vi "Step.GetProperties.vi"(11 "String in":string) -> (1 "Warning":string, 2 "Parameters":dbl[](array[numeric]), 3 "Step":T1)   [LabVIEW 2013, in "Simple Sequence Tools - Shared.lvlib"]
uses:
  Simple Sequence Tools - Shared.lvlib
  Types/Step.Types.ctl
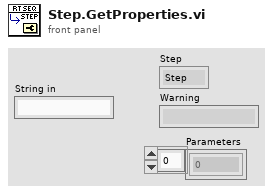
[diagram p1: front panel]
types:
  T1 = typedef "Simple Sequence Tools - Shared.lvlib/Step.Types.ctl" = enum8{"Step", "iStep", "Ramp", "Unchanged", "Unknown", "Sine", "LogSine", "LinearSine", "ForcedRamp", "SquareWave"}
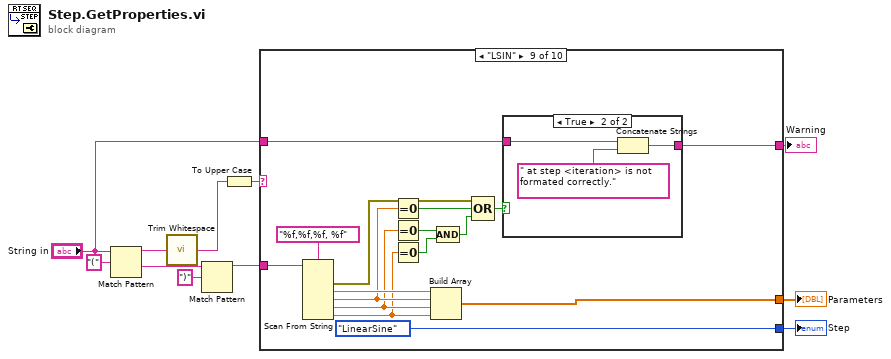
[diagram p0: block diagram]
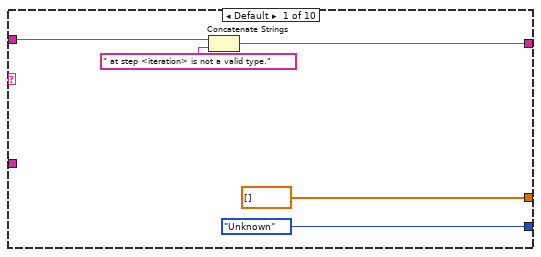
[diagram p2: hidden frame]
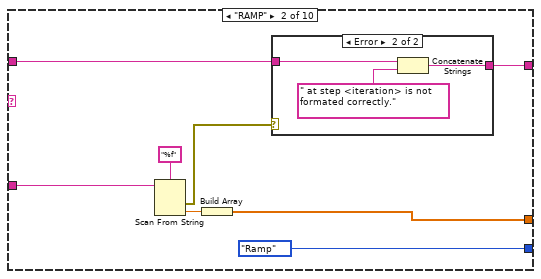
[diagram p3: hidden frame]
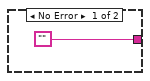
[diagram p4: hidden frame]
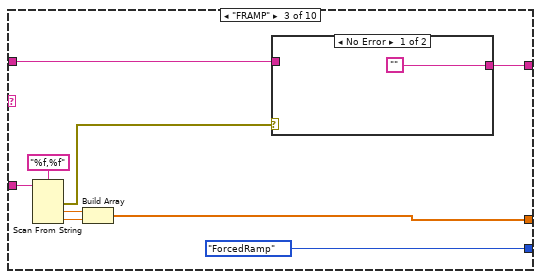
[diagram p5: hidden frame]
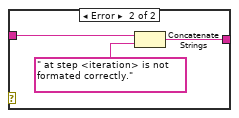
[diagram p6: hidden frame]
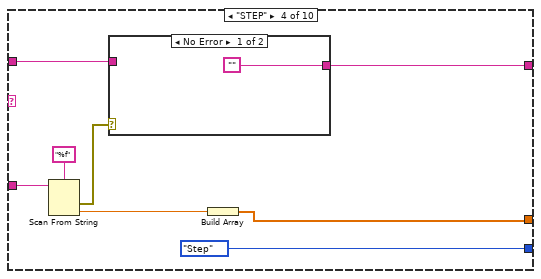
[diagram p7: hidden frame]
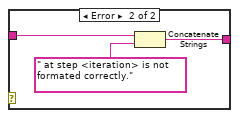
[diagram p8: hidden frame]
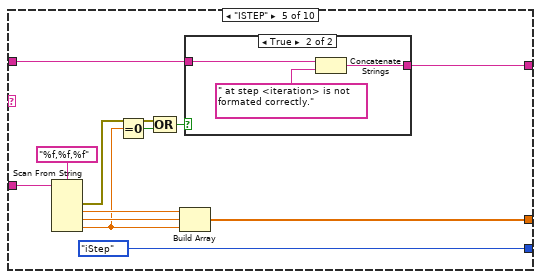
[diagram p9: hidden frame]
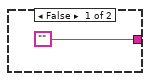
[diagram p10: hidden frame]
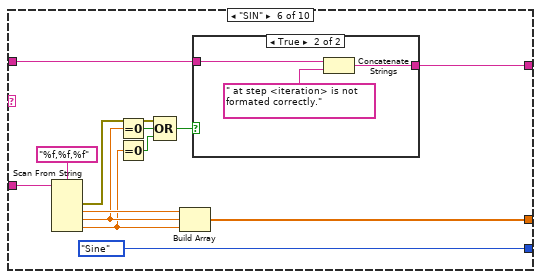
[diagram p11: hidden frame]
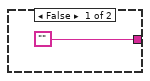
[diagram p12: hidden frame]
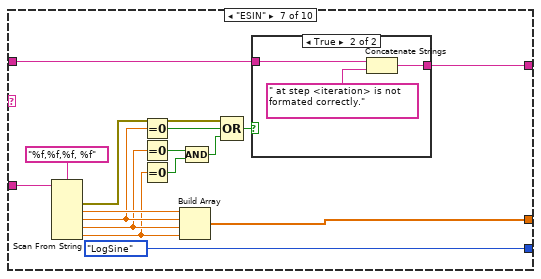
[diagram p13: hidden frame]
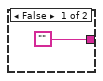
[diagram p14: hidden frame]
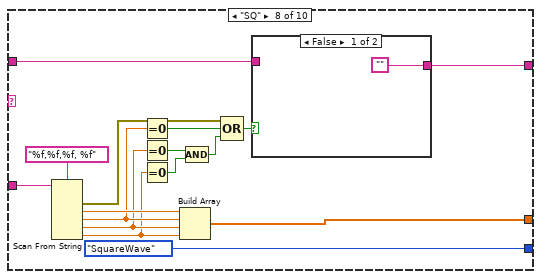
[diagram p15: hidden frame]
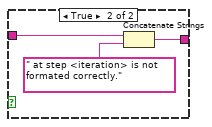
[diagram p16: hidden frame]
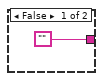
[diagram p17: hidden frame]
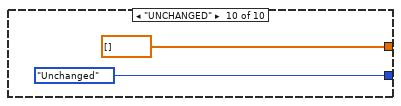
[diagram p18: hidden frame]
diagram:
  n1 = Match Pattern(string="String in", regular expression="(") -> (before substring=w8:string, after substring=w9:string)  [unwired: 1 in, 2 out]
  n2 = call <vilib>:"Trim Whitespace.vi"("string"=w8) -> ("trimmed string"=w11:string)  [unwired: 1 in]
  n3 = Match Pattern(string=w9, regular expression=")") -> (before substring=w4:string)  [unwired: 1 in, 3 out]
  n4 = To Upper Case(1:w11) -> (0:w6:string)
  n5 = case shown="\"LSIN\"" w6 {
    tunnel: [Step.Types."Unknown" Step.Types."Ramp" Step.Types."ForcedRamp" Step.Types."Step" Step.Types."iStep" Step.Types."Sine" Step.Types."LogSine" Step.Types."SquareWave" Step.Types."LinearSine" Step.Types."Unchanged"] -> w5
    tunnel: w4 -> [_ w19 w32 w48 w62 w79 w99 w119 w139 _]
    tunnel: [dbl[] [] w23 w29 w45 w60 w78 w98 w118 w138 dbl[] []] -> w3
    tunnel: "String in" -> [w14 w21 w35 w43 w58 w76 w96 w116 w136 _]
    tunnel: [w12 w20 w34 w42 w57 w75 w95 w115 w135 _] -> w1
    frame Default {
      n6 = Concatenate Strings(w14, " at step <iteration> is not a valid type.") -> (w12:string)
    }
    frame "RAMP" {
      n7 = Scan From String(format string="%f", input string=w19) -> (error out=w22:errorcluster, output 1=w17:dbl)  [unwired: 3 in, 2 out]
      n8 = Build Array(w17) -> (w23:dbl[])
      n9 = case shown="Error" w22 {
        tunnel: w21 -> [_ w27]
        tunnel: ["" w26] -> w20
        frame No Error {
        }
        frame Error {
          n10 = Concatenate Strings(w27, " at step <iteration> is not formated correctly.") -> (w26:string)
        }
      }
    }
    frame "FRAMP" {
      n11 = Scan From String(format string="%f,%f", input string=w32) -> (error out=w36:errorcluster, output 1=w30:dbl, output 2=w31:dbl)  [unwired: 4 in, 2 out]
      n12 = Build Array(w30, w31) -> (w29:dbl[])
      n13 = case shown="No Error" w36 {
        tunnel: w35 -> [_ w40]
        tunnel: ["" w39] -> w34
        frame No Error {
        }
        frame Error {
          n14 = Concatenate Strings(w40, " at step <iteration> is not formated correctly.") -> (w39:string)
        }
      }
    }
    frame "STEP" {
      n15 = Scan From String(format string="%f", input string=w48) -> (error out=w44:errorcluster, output 1=w46:dbl)  [unwired: 3 in, 2 out]
      n16 = case shown="No Error" w44 {
        tunnel: w43 -> [_ w52]
        tunnel: ["" w51] -> w42
        frame No Error {
        }
        frame Error {
          n17 = Concatenate Strings(w52, " at step <iteration> is not formated correctly.") -> (w51:string)
        }
      }
      n18 = Build Array(w46) -> (w45:dbl[])
    }
    frame "ISTEP" {
      n19 = Scan From String(format string="%f,%f,%f", input string=w62) -> (error out=w59:errorcluster, output 1=w63:dbl, output 2=w61:dbl, output 3=w55:dbl)  [unwired: 5 in, 2 out]
      n20 = Equal To 0?(x=w55) -> (x = 0?=w54:bool)
      n21 = Compound Arithmetic op=OR(w59, w54) -> (w56:bool)
      n22 = Build Array(w63, w61, w55) -> (w60:dbl[])
      n23 = case shown="True" w56 {
        tunnel: w58 -> [_ w68]
        tunnel: ["" w67] -> w57
        frame False {
        }
        frame True {
          n24 = Concatenate Strings(w68, " at step <iteration> is not formated correctly.") -> (w67:string)
        }
      }
    }
    frame "SIN" {
      n25 = Scan From String(format string="%f,%f,%f", input string=w79) -> (error out=w77:errorcluster, output 1=w80:dbl, output 2=w72:dbl, output 3=w71:dbl)  [unwired: 5 in, 2 out]
      n26 = Equal To 0?(x=w72) -> (x = 0?=w73:bool)
      n27 = Equal To 0?(x=w71) -> (x = 0?=w70:bool)
      n28 = Compound Arithmetic op=OR(w77, w73, w70) -> (w74:bool)
      n29 = Build Array(w80, w72, w71) -> (w78:dbl[])
      n30 = case shown="True" w74 {
        tunnel: w76 -> [_ w85]
        tunnel: ["" w84] -> w75
        frame False {
        }
        frame True {
          n31 = Concatenate Strings(w85, " at step <iteration> is not formated correctly.") -> (w84:string)
        }
      }
    }
    frame "ESIN" {
      n32 = Scan From String(format string="%f,%f,%f, %f", input string=w99) -> (error out=w97:errorcluster, output 1=w100:dbl, output 2=w92:dbl, output 3=w91:dbl, output 4=w90:dbl)  [unwired: 6 in, 2 out]
      n33 = Equal To 0?(x=w92) -> (x = 0?=w93:bool)
      n34 = Equal To 0?(x=w91) -> (x = 0?=w88:bool)
      n35 = Equal To 0?(x=w90) -> (x = 0?=w89:bool)
      n36 = Build Array(w100, w92, w91, w90) -> (w98:dbl[])
      n37 = Compound Arithmetic op=AND(w88, w89) -> (w87:bool)
      n38 = Compound Arithmetic op=OR(w97, w93, w87) -> (w94:bool)
      n39 = case shown="True" w94 {
        tunnel: w96 -> [_ w105]
        tunnel: ["" w104] -> w95
        frame False {
        }
        frame True {
          n40 = Concatenate Strings(w105, " at step <iteration> is not formated correctly.") -> (w104:string)
        }
      }
    }
    frame "SQ" {
      n41 = Scan From String(format string="%f,%f,%f, %f", input string=w119) -> (error out=w117:errorcluster, output 1=w120:dbl, output 2=w112:dbl, output 3=w111:dbl, output 4=w110:dbl)  [unwired: 6 in, 2 out]
      n42 = Equal To 0?(x=w112) -> (x = 0?=w113:bool)
      n43 = Equal To 0?(x=w111) -> (x = 0?=w108:bool)
      n44 = Equal To 0?(x=w110) -> (x = 0?=w109:bool)
      n45 = Build Array(w120, w112, w111, w110) -> (w118:dbl[])
      n46 = Compound Arithmetic op=AND(w108, w109) -> (w107:bool)
      n47 = Compound Arithmetic op=OR(w117, w113, w107) -> (w114:bool)
      n48 = case shown="False" w114 {
        tunnel: w116 -> [_ w125]
        tunnel: ["" w124] -> w115
        frame False {
        }
        frame True {
          n49 = Concatenate Strings(w125, " at step <iteration> is not formated correctly.") -> (w124:string)
        }
      }
    }
    frame "LSIN" {
      n50 = Scan From String(format string="%f,%f,%f, %f", input string=w139) -> (error out=w137:errorcluster, output 1=w140:dbl, output 2=w132:dbl, output 3=w131:dbl, output 4=w130:dbl)  [unwired: 6 in, 2 out]
      n51 = Equal To 0?(x=w132) -> (x = 0?=w133:bool)
      n52 = Equal To 0?(x=w131) -> (x = 0?=w128:bool)
      n53 = Equal To 0?(x=w130) -> (x = 0?=w129:bool)
      n54 = Build Array(w140, w132, w131, w130) -> (w138:dbl[])
      n55 = Compound Arithmetic op=AND(w128, w129) -> (w127:bool)
      n56 = Compound Arithmetic op=OR(w137, w133, w127) -> (w134:bool)
      n57 = case shown="True" w134 {
        tunnel: w136 -> [_ w145]
        tunnel: ["" w144] -> w135
        frame False {
        }
        frame True {
          n58 = Concatenate Strings(w145, " at step <iteration> is not formated correctly.") -> (w144:string)
        }
      }
    }
    frame "UNCHANGED" {
    }
  }
  "Parameters" <- w3
  "Step" <- w5
  "Warning" <- w1
